vi "Asymmetric RSA Key Testing.vi"() -> ()   [LabVIEW 2021]
uses:
  Key Management/CNG Key Info.ctl
  Asymmetric Encryption/RSA/RSAEncryptionPadding.ctl
  Asymmetric Encryption/dotNET Crypto Asymmetric Encryption.lvlib
  Key Management/dotNET Crypto Key Management.lvlib
panel:
  out "error out":errorcluster
  out "string 2":string
  out "string":string
  out "Private Key":u8[](array[numeric])
  out "Public Key":u8[](array[numeric])
  out "Private Key (Graph) 2":u8[](graph)
  out "Public Key (Graph) 2":u8[](graph)
  out "Key Information 2":T1
  out "Unencrypted":string
  out "Encrypted data out":u8[](array[numeric])
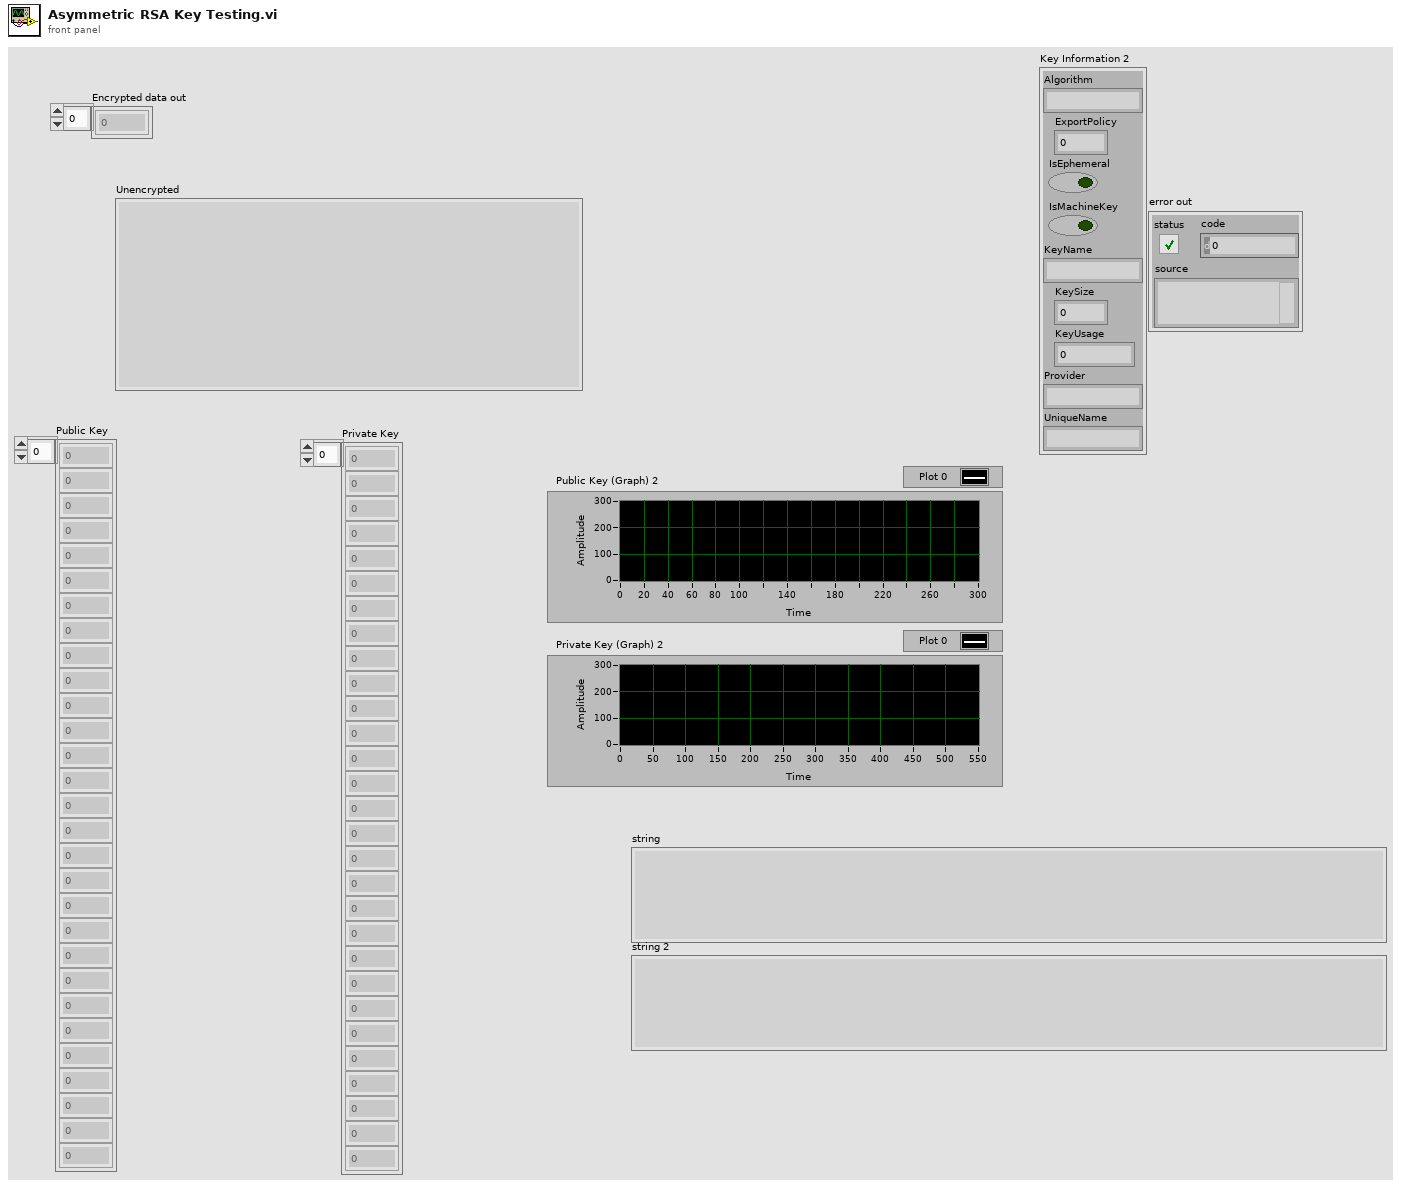
[diagram p1: front panel]
types:
  T1 = typedef "dotNET Crypto Key Management.lvlib/CNG Key Info.ctl" = cluster{"Algorithm":string, "ExportPolicy":i32, "IsEphemeral":bool, "IsMachineKey":bool, "KeyName":string, "KeySize":i32, "KeyUsage":i32, "Provider":string, "UniqueName":string}
  T2 = typedef "dotNET Crypto Asymmetric Encryption.lvlib/RSAEncryptionPadding.ctl" = enum16{"OaepSHA1", "OaepSHA256", "OaepSHA384", "OaepSHA512", "Pkcs1"}
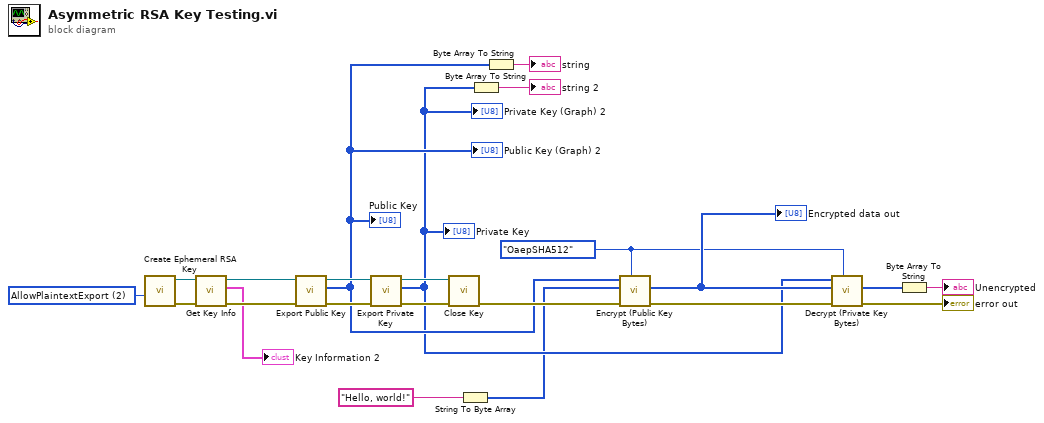
[diagram p0: block diagram]
diagram:
  w12 = 2 items=["None"=0, "AllowExport"=1, "AllowPlaintextExport"=2, "AllowArchiving"=4, "AllowPlaintextArchiving"=8] ("Export Policy (allow export)")
  w21 = RSAEncryptionPadding."OaepSHA512" ("Padding Mode")
  n1 = call "Create Ephemeral RSA Key.vi"("Export Policy (allow export)"=w12) -> ("error out"=w11:errorcluster, "CngKey out"=w10:refnum<k24>)  [unwired: 9 in]
  n2 = call "Get Key Info.vi"("error in (no error)"=w11, "CngKey in"=w10) -> ("error out"=w9:errorcluster, "Key Information"=→"Key Information 2":T1, "CngKey out"=w8:refnum<k24>)  [unwired: 7 in]
  n3 = call "Export Public Key.vi"("error in (no error)"=w9, "CngKey ref in"=w8) -> ("error out"=w20:errorcluster, "Public Key"=w6:u8[], "CngKey ref out"=w18:refnum<k24>)  [unwired: 7 in]
  "Public Key (Graph) 2" <- w6
  "Public Key" <- w6
  n4 = call "Export Private Key.vi"("error in (no error)"=w20, "CngKey ref in"=w18) -> ("error out"=w19:errorcluster, "Private Key"=w3:u8[], "CngKey ref out"=w16:refnum<k24>)  [unwired: 7 in]
  "Private Key (Graph) 2" <- w3
  "Private Key" <- w3
  n5 = call "Close Key.vi"("error in (no error)"=w19, "CngKey in"=w16) -> ("error out"=w17:errorcluster)  [unwired: 9 in]
  n6 = String To Byte Array(string="Hello, world!") -> (unsigned byte array=w1:u8[])
  n7 = Byte Array To String(unsigned byte array=w3) -> (string=→"string 2":string)
  n8 = Byte Array To String(unsigned byte array=w6) -> (string=→"string":string)
  n9 = call "Encrypt (Public Key Bytes).vi"("Padding Mode"=w21, "error in (no error)"=w17, "Raw data in"=w1, "Public key in"=w6) -> ("error out"=w23:errorcluster, "Encrypted data out"=w22:u8[])  [unwired: 6 in]
  "Encrypted data out" <- w22
  n10 = call "Decrypt (Private Key Bytes).vi"("Padding Mode"=w21, "error in (no error)"=w23, "Encrypted data in"=w22, "Private key in"=w3) -> ("error out"=→"error out":errorcluster, "Raw data out"=w14:u8[])  [unwired: 6 in]
  n11 = Byte Array To String(unsigned byte array=w14) -> (string=→"Unencrypted":string)
